vi "new.vi"(8 "Error In":errorcluster, 10 "ref":refnum<vi>, 11 "Generic In":refnum<class "Generic.lvclass">) -> (0 "Error Out":errorcluster, 3 "Generic Out":refnum<class "Generic.lvclass">)   [LabVIEW 2023, in "TLC_Scripto.lvlib" / "Generic.lvclass"]
uses:
  Generic.lvclass
  Generic.lvclass/Generic.ctl
  <userlib>/_OpenG.lib/error/error.llb/openg_error.lvlib
  <vilib>/Utility/Data Type/NI_Data Type.lvlib
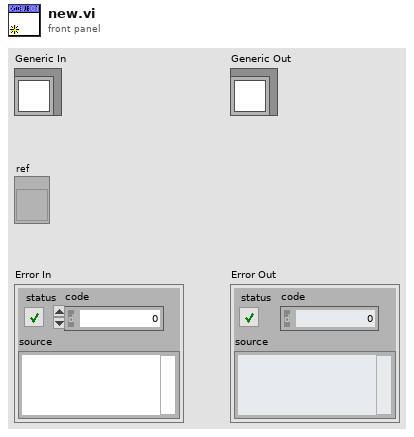
[diagram p1: front panel]
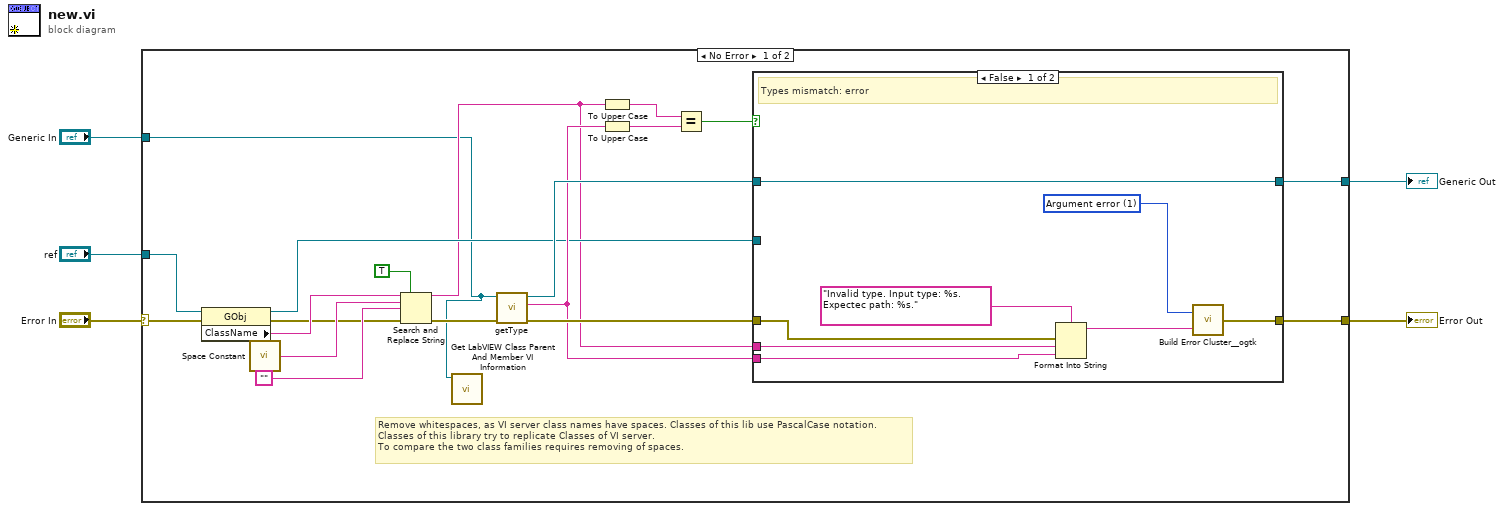
[diagram p0: block diagram]
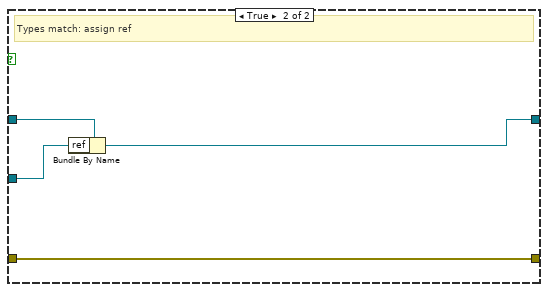
[diagram p2: hidden frame]
diagram:
  n1 = case shown="No Error" "Error In" {
    selector: "Error In" -> [w16 w37]
    tunnel: "Generic In" -> [w6 w38]
    tunnel: [w24 w38] -> w5
    tunnel: "ref" -> [w14 _]
    tunnel: [w20 w37] -> w1
    frame No Error {
      # "Remove whitespaces, as VI server class names have spaces. Classes of this lib use PascalCase notation.\nClasses of this library try to replicate Classes of VI server. \nTo compare the two class families requires removing of spaces."
      n2 = property class="GObj"(reference=w14, error in=w16) -> (reference out=w15:refnum<vi>, error out=w8:errorcluster, "ClassName"=w13:string)
      n3 = call <vilib>:"Space Constant.vi"() -> ("String"=w10:string)
      n4 = Search and Replace String(replace all?=TRUE ("replace all? (F)"), input string=w13, search string=w10, replace string="", error in=w8) -> (result string=w12:string, error out=w7:errorcluster)  [unwired: 3 in, 2 out]
      n5 = call <vilib>:"Get LabVIEW Class Parent And Member VI Information.vi"("variant"=w6) -> ()  [unwired: 7 in, 4 out]
      n6 = call-dynamic "getType.vi"("error in (no error)"=w7, "Generic In"=w6) -> ("error out"=w22:errorcluster, "type"=w19:string, "Generic Out"=w23:refnum<class "Generic.lvclass">)  [unwired: 7 in]
      n7 = To Upper Case(1:w12) -> (0:w18:string)
      n8 = To Upper Case(1:w19) -> (0:w17:string)
      n9 = Equal?(x=w18, y=w17) -> (x = y?=w21:bool)
      n10 = case shown="False" w21 {
        tunnel: [w32 w36] -> w24
        tunnel: w23 -> [w32 w35]
        tunnel: w15 -> [_ w34]
        tunnel: w22 -> [w28 w33]
        tunnel: [w27 w33] -> w20
        tunnel: w19 -> [w26 _]
        tunnel: w12 -> [w25 _]
        frame False {
          w30 = 1 items=["No error", "Argument error", "Memory is full", "Out of zone", "End of file", "File already open", "Generic file I/O error", "File not found", "File permission error", "Disk is full", "Duplicate path", "Too many files open", "System feature not enabled", "Resource file not found", "Cannot add resource", "Resource not found", "Image not found", "Image memory error", "Pen does not exist", "Config type invalid", "Config token not found", "Config parse error", "Config memory error", "Bad external code format", "Bad external code offset", "External code not present", "Null window", "Destroy window error", "Null menu", "Print aborted", "Bad print record", "Print driver error", "Windows error during printing", "Memory error during printing", "Print dialog error", "Generic print error", "Invalid device refnum", "Device not found", "Device parameter error", "Device unit error", "Cannot open device", "Device call aborted", "Generic error", "Cancelled by user", "Object ID too low", "Object ID too high", "Object not in heap", "Unknown heap", "Unknown object (invalid DefProc)", "Unknown object (DefProc not in table)", "Message out of range", "Invalid (null) method", "Unknown message", "Manager call not supported", "Bad address", "Network operation in progress", "Network operation timed out", "Connection is busy", "Network attribute not supported", "Network error", "Address in use", "System out of memory", "Connection aborted", "Connection refused", "Not connected", "Already connected", "Connection closed", "Initialization error (interapplication manager)", "Bad occurrence", "Wait on unbound occurrence handler", "Occurrence queue overflow", "Datalog type conflict", "Unused", "Unrecognized type (interapplication manager)", "Memory corrupt", "Failed to make temporary DLL", "Old CIN version", "Drag socket not found", "Failed to load drop-object", "Failed to register OLE object", "Failed to release OLE object", "Format specifier type mismatch", "Unknown format specifier", "Too few format specifiers", "Too many format specifiers", "Scan failed", "Newer CIN version", "Error converting to variant", "Runtime menu error", "Password tampered", "Variant attribute not found", "Incompatible variant data type", "Event data is not available", "Event Store is not present", "Occurrence is not found", "Event Queue is not created", "Event info is not available", "Refnum passed is NULL", "Error retrieving Class GUID", "Error retrieving CoClass GUID", "Error retrieving TypeLib GUID.", "Bad built application magic bytes.", "Specific driver is different from the specific driver associated with the Logical Name.", "There is no session opened to the class driver.", "Max Error", "MAX - Error with config objects", "MAX - Error loading configuration", "MAX - Group not supported"]
          # "Types mismatch: error"
          n11 = Format Into String(format string="Invalid type. Input type: %s. Expectec path: %s.", error in=w28, w25, w26) -> (resulting string=w31:string)  [unwired: 1 in, 1 out]
          n12 = call <userlib>:"Build Error Cluster__ogtk.vi"("String to Prepend to source (\"\")"=w31, "code"=w30) -> ("error out"=w27:errorcluster)
        }
        frame True {
          # "Types match: assign ref"
          n13 = Bundle By Name(cluster=w35, "ref"=w34) -> (w36:refnum<class "Generic.lvclass">)
        }
      }
    }
    frame Error {
    }
  }
  "Generic Out" <- w5
  "Error Out" <- w1
